vi "connect.vi"(8 "error in (no error)":errorcluster, 11 "tcpDevice in":refnum<class "tcpDevice.lvclass">) -> (0 "error out":errorcluster, 3 "tcpDevice out":refnum<class "tcpDevice.lvclass">)   [LabVIEW 2016, in "tcpDevice.lvclass"]
uses:
  tcpDevice.lvclass
  tcpDevice.lvclass/tcpDevice.ctl
  ts_labview_tcp/TCPClient/TCPClient.lvclass
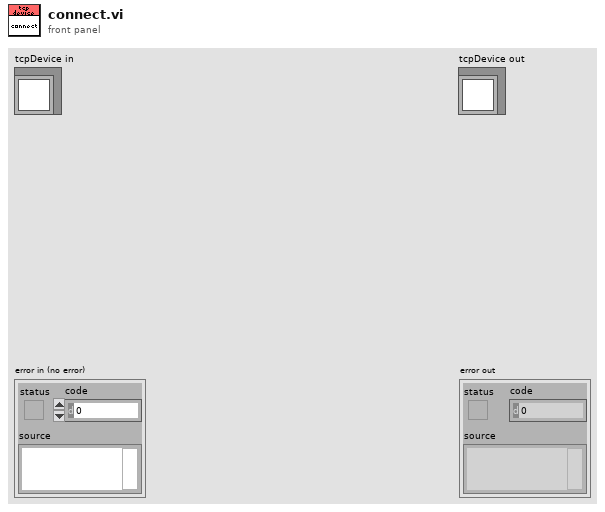
[diagram p1: front panel]
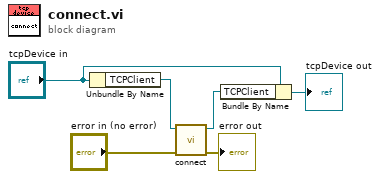
[diagram p0: block diagram]
diagram:
  n1 = Unbundle By Name("tcpDevice in") -> ("TCPClient"=w6:refnum<class "TCPClient.lvclass">)
  n2 = call-dynamic "connect.vi"("error in (no error)"="error in (no error)", "TCPClient in"=w6) -> ("error out"=→"error out":errorcluster, "TCPClient out"=w4:refnum<class "TCPClient.lvclass">)  [unwired: 8 in]
  n3 = Bundle By Name(cluster="tcpDevice in", "TCPClient"=w4) -> (→"tcpDevice out":refnum<class "tcpDevice.lvclass">)
